vi "Read Coils.vi"(8 "error in (no error)":errorcluster, 9 "number of coils":u16, 10 "starting address":u16, 11 "Modbus master in":refnum<class "Modbus Master.lvclass">) -> (0 "error out":errorcluster, 2 "coil values":bool[](array[boolean]), 3 "Modbus master out":refnum<class "Modbus Master.lvclass">)   [LabVIEW 2021, in "Modbus Master.lvclass"]
doc: "Reads values from contiguous coils. The maximum number of coils this VI can read is 2,000."
uses:
  Modbus Master.lvclass
  Modbus Master.lvclass/Modbus Master.ctl
  Modbus Data Unit/Modbus Data Unit.lvclass/Modbus Data Unit.ctl
  Network Protocol/Network Master/Network Master.lvclass/Network Master.ctl
  Master Function Definition/Read Coils Request.vi
  Network Protocol/Network Master/Read write Master.vi
  Master Function Definition/Read Coils Response.vi
  Modbus Data Unit/Construct PDU.vi
  Utility/Bytes to Bits.vi
  Data Model/Error Generator.vi
  Master Function Definition/Function code mismatch error.vi
  Modbus Data Unit/Deconstruct PDU.vi
  Modbus Data Unit/Modbus Data Unit.lvclass
  Transmission Data Unit/Transmission Data Unit.lvclass
  Network Protocol/Network Master/Network Master.lvclass
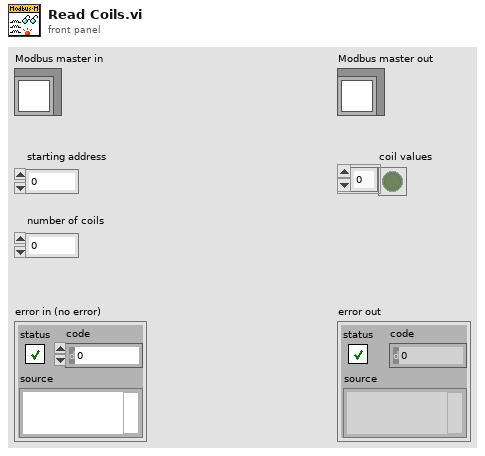
[diagram p1: front panel]
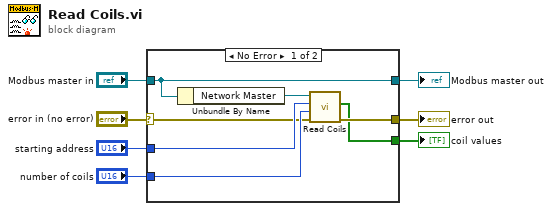
[diagram p0: block diagram]
diagram:
  n1 = case shown="No Error" "error in (no error)" {
    selector: "error in (no error)" -> [w8 w16]
    tunnel: [w14 w16] -> w5
    tunnel: [w9 w15] -> w6
    tunnel: "Modbus master in" -> [w9 w15]
    tunnel: "starting address" -> [w12 _]
    tunnel: "number of coils" -> [w11 _]
    tunnel: [w13 _] -> w4
    frame No Error {
      n2 = Unbundle By Name(w9) -> ("Network Master"=w10:refnum<class "Network Master.lvclass">)
      n3 = call "Read Coils.vi"("error in (no error)"=w8, "number of coils"=w11, "starting address"=w12, "Modbus master in"=w10) -> ("error out"=w14:errorcluster, "coil values"=w13:bool[])  [unwired: 5 in, 1 out]
    }
    frame Error {
    }
  }
  "error out" <- w5
  "Modbus master out" <- w6
  "coil values" <- w4
